vi "Analog read.vi"(0 "VISA Refnum in":refnum<visa-resource-name>, 1 "error in (no error)":errorcluster) -> (2 "VISA Refnum out":refnum<visa-resource-name>, 3 "Numeric":dbl, 4 "error out":errorcluster)   [LabVIEW 2014]
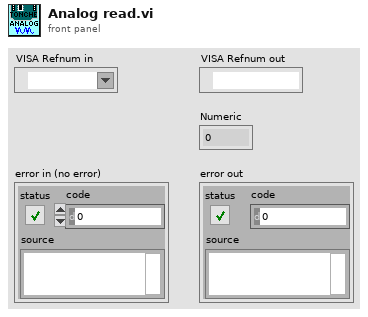
[diagram p1: front panel]
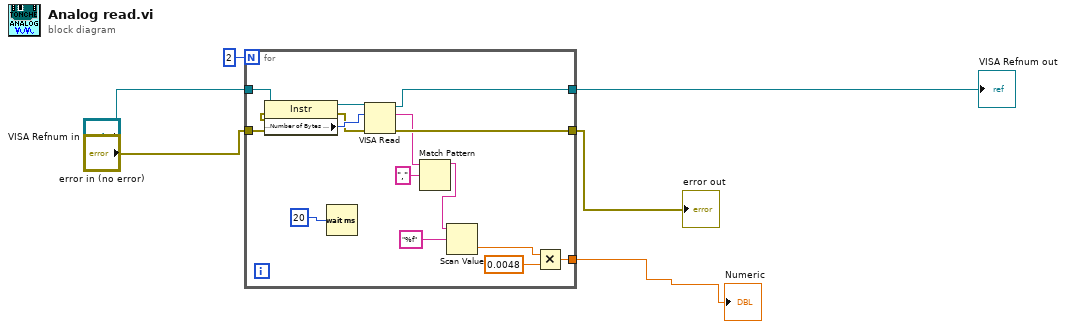
[diagram p0: block diagram]
diagram:
  n1 = for {
    N: 2 -> [_]
    tunnel: "error in (no error)" -> [w20]
    tunnel: [w19] -> w3
    tunnel: "VISA Refnum in" -> [w21]
    tunnel: [w18] -> w4
    tunnel: [w7] -> w6
    n2 = property class="Instr"(reference=w21, error in=w20) -> (reference out=w15:refnum<visa-resource-name>, error out=w14:errorcluster, "Serial Settings:Number of Bytes at Serial Port"=w16:u32)
    n3 = Wait (ms)(milliseconds to wait=u32 20) -> ()  [unwired: 1 out]
    n4 = VISA Read(VISA resource name=w15, byte count=w16, error in (no error)=w14) -> (VISA resource name out=w18:refnum<visa-resource-name>, read buffer=w13:string, error out=w19:errorcluster)  [unwired: 1 out]
    n5 = Match Pattern(string=w13, regular expression=",") -> (before substring=w11:string)  [unwired: 1 in, 3 out]
    n6 = Scan Value(string=w11, format string="%f") -> (value=w8:dbl)  [unwired: 1 in, 1 out]
    n7 = Multiply(x=w8, y=0.0048) -> (x*y=w7:dbl)
  }
  "Numeric" <- w6
  "VISA Refnum out" <- w4
  "error out" <- w3
